vi "CRYUnflatten Calibration 2D.vi"(11 "Flattened Calibration":string) -> (0 "Error?":bool=TRUE, 2 "Calibration Step Out":T1 {"Calibration 2D"."Sens Curve"."Z data" items=["dB", "Lin"]; "Calibration 2D"."Sens Curve"."X data" items=["dB", "Lin"]; "Calibration 2D"."Sens Curve"."Y data" items=["dB", "Lin"]; "Calibration 2D"."Sens Curve"."Z dB ref" format="%.1f"; "Calibration 2D"."Sens Curve"."Z axis" items=["Log", "Lin"]; "Calibration 2D"."Sens Curve"."X dB ref" format="%.1f"; "Calibration 2D"."Sens Curve"."X axis" items=["Log", "Lin"]; "Calibration 2D"."Sens Curve"."Y axis" items=["Log", "Lin"]; "Calibration 2D"."Sens Curve"."Y dB ref" format="%.1f"; "Calibration 2D"."Sens Curve"."Curve"."z" format="%.2f"; "Calibration 2D"."Sens Curve"."Curve"."y" format="%.2f"; "Calibration 2D"."Sens Curve"."Curve"."x" format="%.2f"; "Calibration 2D"."EQ Curve"."Z data" items=["dB", "Lin"]; "Calibration 2D"."EQ Curve"."X data" items=["dB", "Lin"]; "Calibration 2D"."EQ Curve"."Y data" items=["dB", "Lin"]; "Calibration 2D"."EQ Curve"."Z dB ref" format="%.1f"; "Calibration 2D"."EQ Curve"."Z axis" items=["Log", "Lin"]; "Calibration 2D"."EQ Curve"."X dB ref" format="%.1f"; "Calibration 2D"."EQ Curve"."X axis" items=["Log", "Lin"]; "Calibration 2D"."EQ Curve"."Y axis" items=["Log", "Lin"]; "Calibration 2D"."EQ Curve"."Y dB ref" format="%.1f"; "Calibration 2D"."EQ Curve"."Curve"."z" format="%.2f"; "Calibration 2D"."EQ Curve"."Curve"."y" format="%.2f"; "Calibration 2D"."EQ Curve"."Curve"."x" format="%.2f"; "Calibration 2D"."Corr Curve"."Z data" items=["dB", "Lin"]; "Calibration 2D"."Corr Curve"."X data" items=["dB", "Lin"]; "Calibration 2D"."Corr Curve"."Y data" items=["dB", "Lin"]; "Calibration 2D"."Corr Curve"."Z dB ref" format="%.1f"; "Calibration 2D"."Corr Curve"."Z axis" items=["Log", "Lin"]; "Calibration 2D"."Corr Curve"."X dB ref" format="%.1f"; "Calibration 2D"."Corr Curve"."X axis" items=["Log", "Lin"]; "Calibration 2D"."Corr Curve"."Y axis" items=["Log", "Lin"]; "Calibration 2D"."Corr Curve"."Y dB ref" format="%.1f"; "Calibration 2D"."Corr Curve"."Curve"."z" format="%.2f"; "Calibration 2D"."Corr Curve"."Curve"."y" format="%.2f"; "Calibration 2D"."Corr Curve"."Curve"."x" format="%.2f"; "Calibration 2D"."Calibration"."EQ Step size" items=["R10", "R20", "R40", "R80", "User"]; "Calibration 2D"."Calibration"."Corr Step size" items=["R10", "R20", "R40", "R80", "User"]}, 3 "Header info":T5={"Data type"="Data            ", "Version"=1, "Dimensions"=0})   [LabVIEW 2013]
uses:
  Typedef Control/CRYCalibration All Cluster.ctl
  Typedef Control/CRYCalibration 2DCluster.ctl
  Typedef Control/CRYCalibration Cluster.ctl
  Typedef Control/CRYData Cluster.ctl
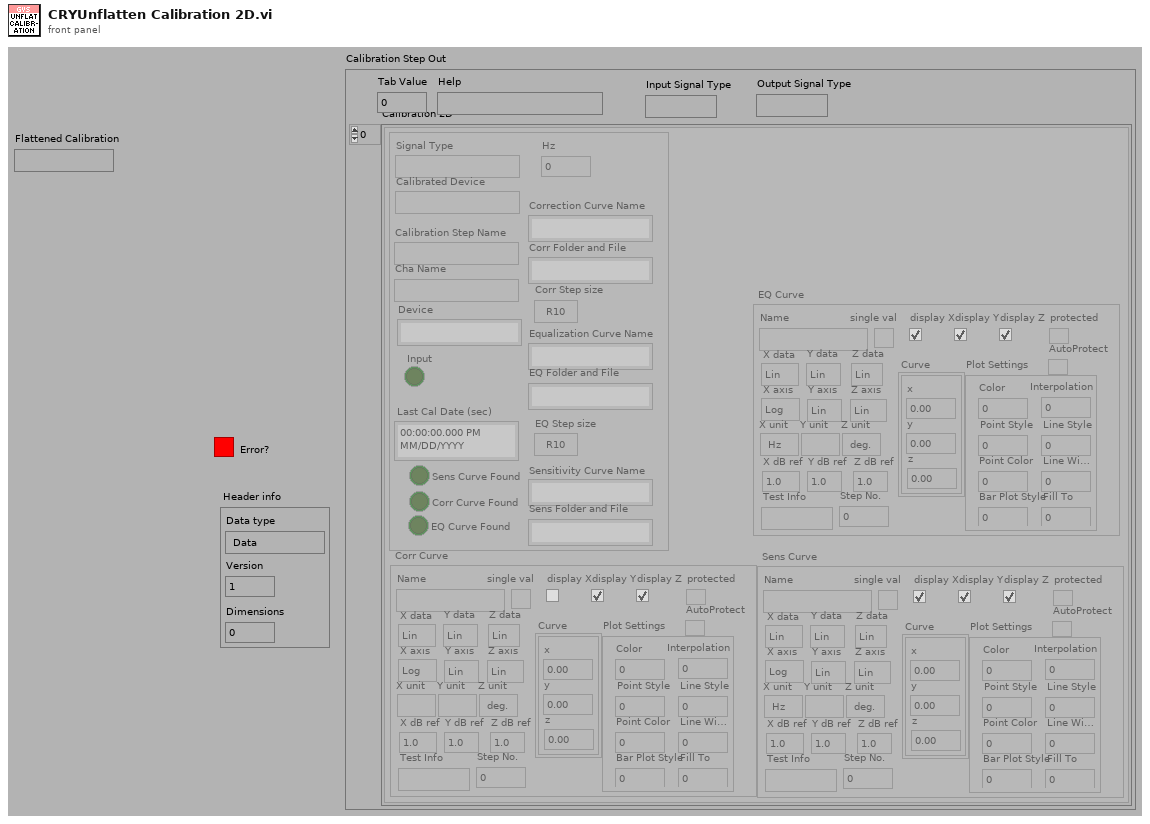
[diagram p1: front panel]
types:
  T1 = typedef "CRYCalibration All Cluster.ctl" = cluster{"Calibration 2D":T2[], "Help":string, "Tab Value":i32, "Input Signal Type":string, "Output Signal Type":string}
  T2 = typedef "CRYCalibration 2DCluster.ctl" = cluster{"Calibration":T3, "Corr Curve":T4, "EQ Curve":T4, "Sens Curve":T4}
  T3 = typedef "CRYCalibration Cluster.ctl" = cluster{"Calibration Step Name":string, "Device":string, "Correction Curve Name":string, "Equalization Curve Name":string, "Sensitivity Curve Name":string, "Corr Folder and File":string, "EQ Folder and File":string, "Sens Folder and File":string, "Corr Step size":u16, "EQ Step size":u16, "Input":bool, "Last Cal Date (sec)":timestamp, "Cha Name":string, "Corr Curve Found":bool, "EQ Curve Found":bool, "Sens Curve Found":bool, "Signal Type":string, "Calibrated Device":string, "Hz":u32}
  T4 = typedef "CRYData Cluster.ctl" = cluster{"Name":string, "Curve":cluster{"x":dbl, "y":dbl, "z":dbl}[], "X data":u16, "Y data":u16, "Z data":u16, "X axis":u16, "Y axis":u16, "Z axis":u16, "X unit":string, "Y unit":string, "Z unit":string, "X dB ref":dbl, "Y dB ref":dbl, "Z dB ref":dbl, "single val":bool, "protected":bool, "display X":bool, "display Y":bool, "display Z":bool, "Test Info":string, "Step No.":i32, "Plot Settings":cluster{"Color":u32, "Interpolation":u8, "Point Style":u8, "Line Style":u8, "Point Color":u32, "Line Width":u8, "Bar Plot Style":u8, "Fill To":i16}, "AutoProtect":bool}
  T5 = cluster{"Data type":string, "Version":u16, "Dimensions":u8}
  T6 = cluster{"Calibration":cluster{"Calibration":cluster{"Calibration Step Name":string, "Last Ch":i32, "Device":string, "Correction Curve Name":string, "Equalization Curve Name":string, "Sensitivity Curve Name":string, "Corr Folder and File":string, "EQ Folder and File":string, "Sens Folder and File":string, "Corr Step size":u16, "EQ Step size":u16, "Input":bool, "Last Cal Date (sec)":timestamp, "Chan Name":string, "Corr Curve Found":bool, "EQ Curve Found":bool, "Sens Curve Found":bool}, "Corr Curve":cluster{"Name":string, "Curve":cluster{"x":dbl, "y":dbl, "z":dbl}[], "X data":u16, "Y data":u16, "Z data":u16, "X axis":u16, "Y axis":u16, "Z axis":u16, "X unit":string, "Y unit":string, "Z unit":string, "X dB ref":dbl, "Y dB ref":dbl, "Z dB ref":dbl, "single val":bool, "protected":bool, "display X":bool, "display Y":bool, "display Z":bool, "Test Info":string, "Step No.":u16, "Plot Settings":cluster{"Color":u32, "Interpolation":u8, "Point Style":u8, "Line Style":u8, "Point Color":u32, "Line Width":u8, "Bar Plot Style":u8, "Fill To":i16}, "AutoProtect":bool}, "EQ Curve":cluster{"Name":string, "Curve":cluster{"x":dbl, "y":dbl, "z":dbl}[], "X data":u16, "Y data":u16, "Z data":u16, "X axis":u16, "Y axis":u16, "Z axis":u16, "X unit":string, "Y unit":string, "Z unit":string, "X dB ref":dbl, "Y dB ref":dbl, "Z dB ref":dbl, "single val":bool, "protected":bool, "display X":bool, "display Y":bool, "display Z":bool, "Test Info":string, "Step No.":u16, "Plot Settings":cluster{"Color":u32, "Interpolation":u8, "Point Style":u8, "Line Style":u8, "Point Color":u32, "Line Width":u8, "Bar Plot Style":u8, "Fill To":i16}, "AutoProtect":bool}, "Sens Curve":cluster{"Name":string, "Curve":cluster{"x":dbl, "y":dbl, "z":dbl}[], "X data":u16, "Y data":u16, "Z data":u16, "X axis":u16, "Y axis":u16, "Z axis":u16, "X unit":string, "Y unit":string, "Z unit":string, "X dB ref":dbl, "Y dB ref":dbl, "Z dB ref":dbl, "single val":bool, "protected":bool, "display X":bool, "display Y":bool, "display Z":bool, "Test Info":string, "Step No.":u16, "Plot Settings":cluster{"Color":u32, "Interpolation":u8, "Point Style":u8, "Line Style":u8, "Point Color":u32, "Line Width":u8, "Bar Plot Style":u8, "Fill To":i16}, "AutoProtect":bool}}[], "Help":string, "Tab Value":i32}
  T7 = cluster{"Calibration 2D":cluster{"Calibration":cluster{"Calibration Step Name":string, "Last Ch":i32, "Device":string, "Correction Curve Name":string, "Equalization Curve Name":string, "Sensitivity Curve Name":string, "Corr Folder and File":string, "EQ Folder and File":string, "Sens Folder and File":string, "Corr Step size":u16, "EQ Step size":u16, "Input":bool, "Last Cal Date (sec)":timestamp, "Cha Name":string, "Corr Curve Found":bool, "EQ Curve Found":bool, "Sens Curve Found":bool}, "Corr Curve":cluster{"Name":string, "Curve":cluster{"x":dbl, "y":dbl, "z":dbl}[], "X data":u16, "Y data":u16, "Z data":u16, "X axis":u16, "Y axis":u16, "Z axis":u16, "X unit":string, "Y unit":string, "Z unit":string, "X dB ref":dbl, "Y dB ref":dbl, "Z dB ref":dbl, "single val":bool, "protected":bool, "display X":bool, "display Y":bool, "display Z":bool, "Test Info":string, "Step No.":i32, "Plot Settings":cluster{"Color":u32, "Interpolation":u8, "Point Style":u8, "Line Style":u8, "Point Color":u32, "Line Width":u8, "Bar Plot Style":u8, "Fill To":i16}, "AutoProtect":bool}, "EQ Curve":cluster{"Name":string, "Curve":cluster{"x":dbl, "y":dbl, "z":dbl}[], "X data":u16, "Y data":u16, "Z data":u16, "X axis":u16, "Y axis":u16, "Z axis":u16, "X unit":string, "Y unit":string, "Z unit":string, "X dB ref":dbl, "Y dB ref":dbl, "Z dB ref":dbl, "single val":bool, "protected":bool, "display X":bool, "display Y":bool, "display Z":bool, "Test Info":string, "Step No.":i32, "Plot Settings":cluster{"Color":u32, "Interpolation":u8, "Point Style":u8, "Line Style":u8, "Point Color":u32, "Line Width":u8, "Bar Plot Style":u8, "Fill To":i16}, "AutoProtect":bool}, "Sens Curve":cluster{"Name":string, "Curve":cluster{"x":dbl, "y":dbl, "z":dbl}[], "X data":u16, "Y data":u16, "Z data":u16, "X axis":u16, "Y axis":u16, "Z axis":u16, "X unit":string, "Y unit":string, "Z unit":string, "X dB ref":dbl, "Y dB ref":dbl, "Z dB ref":dbl, "single val":bool, "protected":bool, "display X":bool, "display Y":bool, "display Z":bool, "Test Info":string, "Step No.":i32, "Plot Settings":cluster{"Color":u32, "Interpolation":u8, "Point Style":u8, "Line Style":u8, "Point Color":u32, "Line Width":u8, "Bar Plot Style":u8, "Fill To":i16}, "AutoProtect":bool}}[], "Help":string, "Tab Value":i32}
  T8 = cluster{"unsigned byte array[0]":u8, "unsigned byte array[1]":u8, "unsigned byte array[2]":u8}
  T9 = cluster{"Calibration":cluster{"Calibration Step Name":string, "Last Ch":i32, "Device":string, "Correction Curve Name":string, "Equalization Curve Name":string, "Sensitivity Curve Name":string, "Corr Folder and File":string, "EQ Folder and File":string, "Sens Folder and File":string, "Corr Step size":u16, "EQ Step size":u16, "Input":bool, "Last Cal Date (sec)":timestamp, "Chan Name":string, "Corr Curve Found":bool, "EQ Curve Found":bool, "Sens Curve Found":bool}, "Corr Curve":cluster{"Name":string, "Curve":cluster{"x":dbl, "y":dbl, "z":dbl}[], "X data":u16, "Y data":u16, "Z data":u16, "X axis":u16, "Y axis":u16, "Z axis":u16, "X unit":string, "Y unit":string, "Z unit":string, "X dB ref":dbl, "Y dB ref":dbl, "Z dB ref":dbl, "single val":bool, "protected":bool, "display X":bool, "display Y":bool, "display Z":bool, "Test Info":string, "Step No.":u16, "Plot Settings":cluster{"Color":u32, "Interpolation":u8, "Point Style":u8, "Line Style":u8, "Point Color":u32, "Line Width":u8, "Bar Plot Style":u8, "Fill To":i16}, "AutoProtect":bool}, "EQ Curve":cluster{"Name":string, "Curve":cluster{"x":dbl, "y":dbl, "z":dbl}[], "X data":u16, "Y data":u16, "Z data":u16, "X axis":u16, "Y axis":u16, "Z axis":u16, "X unit":string, "Y unit":string, "Z unit":string, "X dB ref":dbl, "Y dB ref":dbl, "Z dB ref":dbl, "single val":bool, "protected":bool, "display X":bool, "display Y":bool, "display Z":bool, "Test Info":string, "Step No.":u16, "Plot Settings":cluster{"Color":u32, "Interpolation":u8, "Point Style":u8, "Line Style":u8, "Point Color":u32, "Line Width":u8, "Bar Plot Style":u8, "Fill To":i16}, "AutoProtect":bool}, "Sens Curve":cluster{"Name":string, "Curve":cluster{"x":dbl, "y":dbl, "z":dbl}[], "X data":u16, "Y data":u16, "Z data":u16, "X axis":u16, "Y axis":u16, "Z axis":u16, "X unit":string, "Y unit":string, "Z unit":string, "X dB ref":dbl, "Y dB ref":dbl, "Z dB ref":dbl, "single val":bool, "protected":bool, "display X":bool, "display Y":bool, "display Z":bool, "Test Info":string, "Step No.":u16, "Plot Settings":cluster{"Color":u32, "Interpolation":u8, "Point Style":u8, "Line Style":u8, "Point Color":u32, "Line Width":u8, "Bar Plot Style":u8, "Fill To":i16}, "AutoProtect":bool}}[]
  T10 = cluster{"Calibration Step Name":string, "Last Ch":i32, "Device":string, "Correction Curve Name":string, "Equalization Curve Name":string, "Sensitivity Curve Name":string, "Corr Folder and File":string, "EQ Folder and File":string, "Sens Folder and File":string, "Corr Step size":u16, "EQ Step size":u16, "Input":bool, "Last Cal Date (sec)":timestamp, "Chan Name":string, "Corr Curve Found":bool, "EQ Curve Found":bool, "Sens Curve Found":bool}
  T11 = cluster{"Name":string, "Curve":cluster{"x":dbl, "y":dbl, "z":dbl}[], "X data":u16, "Y data":u16, "Z data":u16, "X axis":u16, "Y axis":u16, "Z axis":u16, "X unit":string, "Y unit":string, "Z unit":string, "X dB ref":dbl, "Y dB ref":dbl, "Z dB ref":dbl, "single val":bool, "protected":bool, "display X":bool, "display Y":bool, "display Z":bool, "Test Info":string, "Step No.":u16, "Plot Settings":cluster{"Color":u32, "Interpolation":u8, "Point Style":u8, "Line Style":u8, "Point Color":u32, "Line Width":u8, "Bar Plot Style":u8, "Fill To":i16}, "AutoProtect":bool}
  T12 = cluster{"Calibration":cluster{"Calibration Step Name":string, "Last Ch":i32, "Device":string, "Correction Curve Name":string, "Equalization Curve Name":string, "Sensitivity Curve Name":string, "Corr Folder and File":string, "EQ Folder and File":string, "Sens Folder and File":string, "Corr Step size":u16, "EQ Step size":u16, "Input":bool, "Last Cal Date (sec)":timestamp, "Cha Name":string, "Corr Curve Found":bool, "EQ Curve Found":bool, "Sens Curve Found":bool}, "Corr Curve":cluster{"Name":string, "Curve":cluster{"x":dbl, "y":dbl, "z":dbl}[], "X data":u16, "Y data":u16, "Z data":u16, "X axis":u16, "Y axis":u16, "Z axis":u16, "X unit":string, "Y unit":string, "Z unit":string, "X dB ref":dbl, "Y dB ref":dbl, "Z dB ref":dbl, "single val":bool, "protected":bool, "display X":bool, "display Y":bool, "display Z":bool, "Test Info":string, "Step No.":i32, "Plot Settings":cluster{"Color":u32, "Interpolation":u8, "Point Style":u8, "Line Style":u8, "Point Color":u32, "Line Width":u8, "Bar Plot Style":u8, "Fill To":i16}, "AutoProtect":bool}, "EQ Curve":cluster{"Name":string, "Curve":cluster{"x":dbl, "y":dbl, "z":dbl}[], "X data":u16, "Y data":u16, "Z data":u16, "X axis":u16, "Y axis":u16, "Z axis":u16, "X unit":string, "Y unit":string, "Z unit":string, "X dB ref":dbl, "Y dB ref":dbl, "Z dB ref":dbl, "single val":bool, "protected":bool, "display X":bool, "display Y":bool, "display Z":bool, "Test Info":string, "Step No.":i32, "Plot Settings":cluster{"Color":u32, "Interpolation":u8, "Point Style":u8, "Line Style":u8, "Point Color":u32, "Line Width":u8, "Bar Plot Style":u8, "Fill To":i16}, "AutoProtect":bool}, "Sens Curve":cluster{"Name":string, "Curve":cluster{"x":dbl, "y":dbl, "z":dbl}[], "X data":u16, "Y data":u16, "Z data":u16, "X axis":u16, "Y axis":u16, "Z axis":u16, "X unit":string, "Y unit":string, "Z unit":string, "X dB ref":dbl, "Y dB ref":dbl, "Z dB ref":dbl, "single val":bool, "protected":bool, "display X":bool, "display Y":bool, "display Z":bool, "Test Info":string, "Step No.":i32, "Plot Settings":cluster{"Color":u32, "Interpolation":u8, "Point Style":u8, "Line Style":u8, "Point Color":u32, "Line Width":u8, "Bar Plot Style":u8, "Fill To":i16}, "AutoProtect":bool}}[]
  T13 = cluster{"Calibration Step Name":string, "Last Ch":i32, "Device":string, "Correction Curve Name":string, "Equalization Curve Name":string, "Sensitivity Curve Name":string, "Corr Folder and File":string, "EQ Folder and File":string, "Sens Folder and File":string, "Corr Step size":u16, "EQ Step size":u16, "Input":bool, "Last Cal Date (sec)":timestamp, "Cha Name":string, "Corr Curve Found":bool, "EQ Curve Found":bool, "Sens Curve Found":bool}
  T14 = cluster{"Name":string, "Curve":cluster{"x":dbl, "y":dbl, "z":dbl}[], "X data":u16, "Y data":u16, "Z data":u16, "X axis":u16, "Y axis":u16, "Z axis":u16, "X unit":string, "Y unit":string, "Z unit":string, "X dB ref":dbl, "Y dB ref":dbl, "Z dB ref":dbl, "single val":bool, "protected":bool, "display X":bool, "display Y":bool, "display Z":bool, "Test Info":string, "Step No.":i32, "Plot Settings":cluster{"Color":u32, "Interpolation":u8, "Point Style":u8, "Line Style":u8, "Point Color":u32, "Line Width":u8, "Bar Plot Style":u8, "Fill To":i16}, "AutoProtect":bool}
  T15 = cluster{"substring":string, u16, "unsigned byte array[2]":u8}
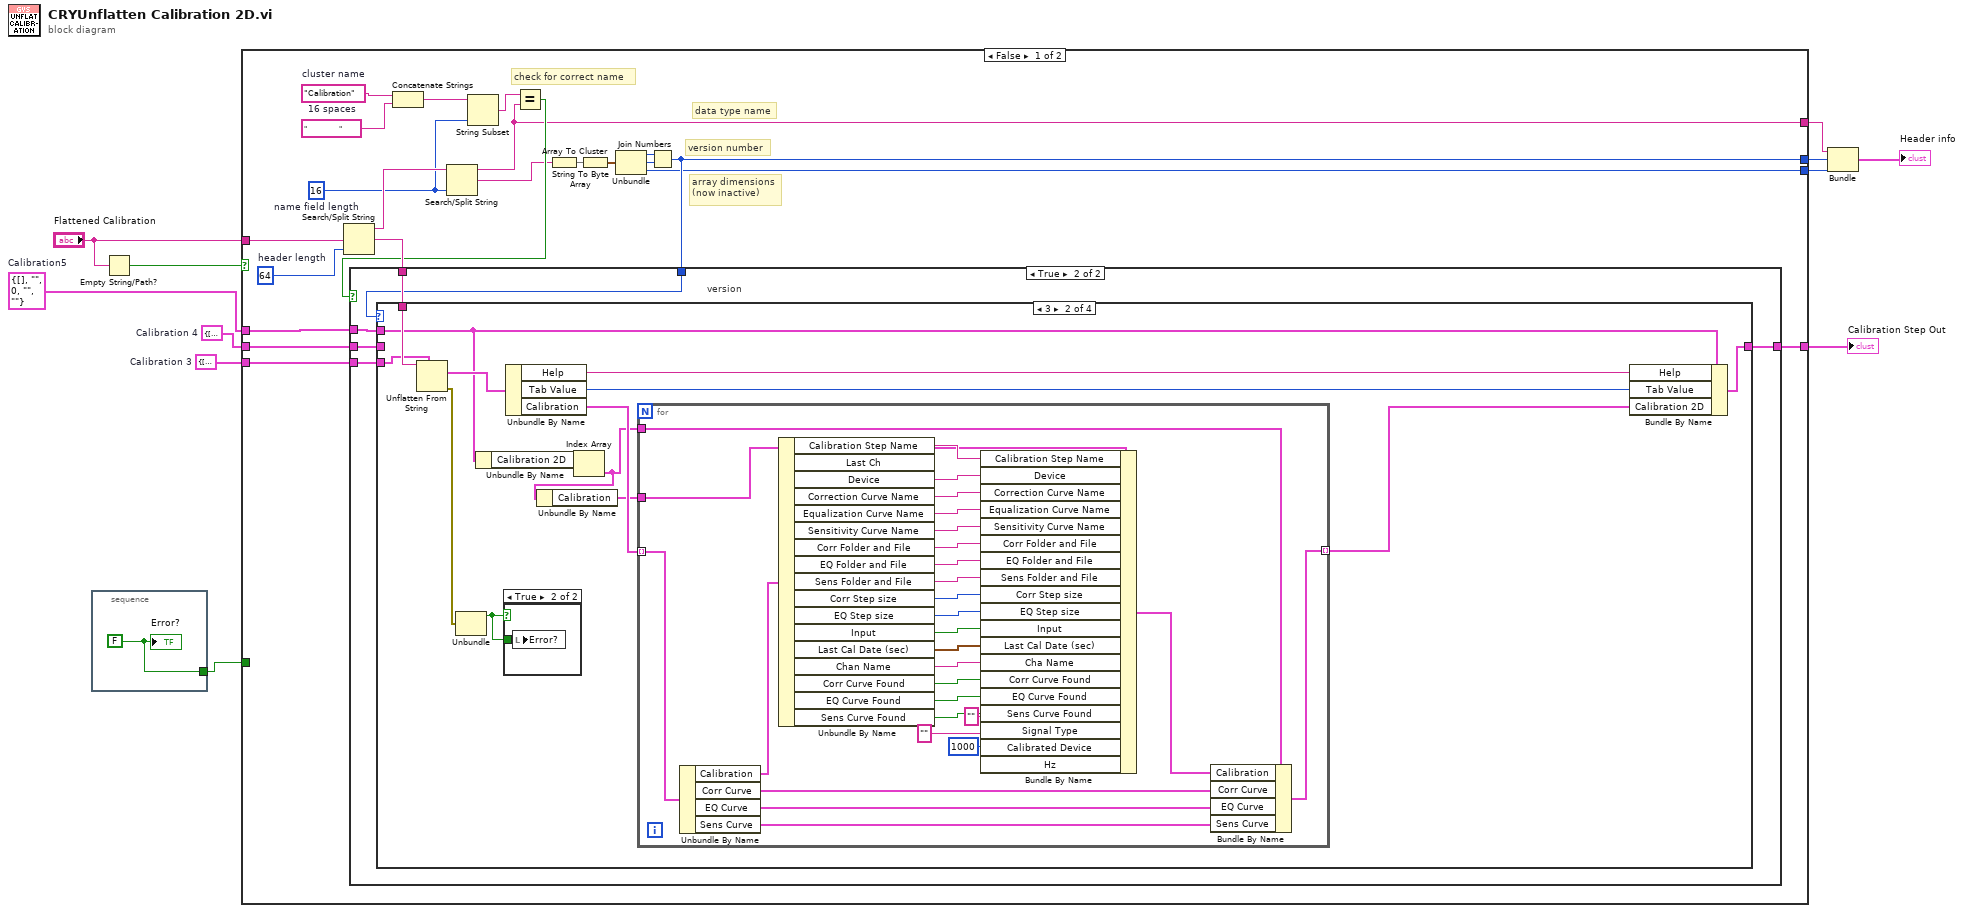
[diagram p0: block diagram]
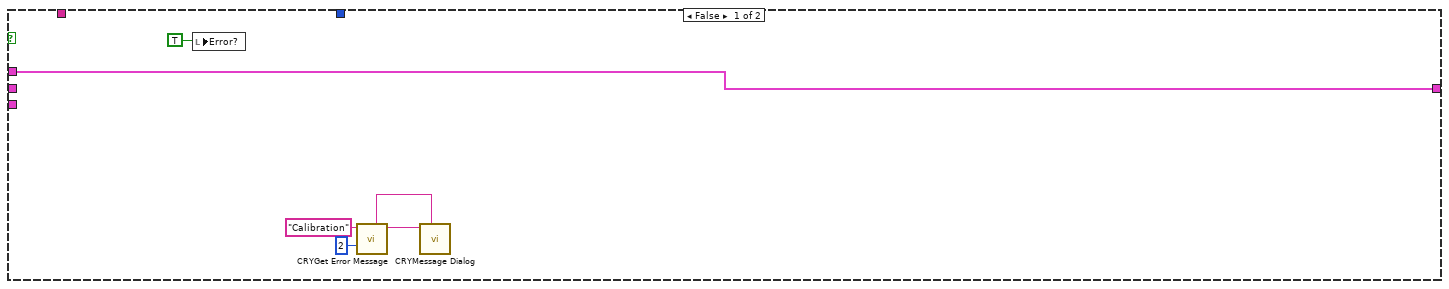
[diagram p2: hidden frame]
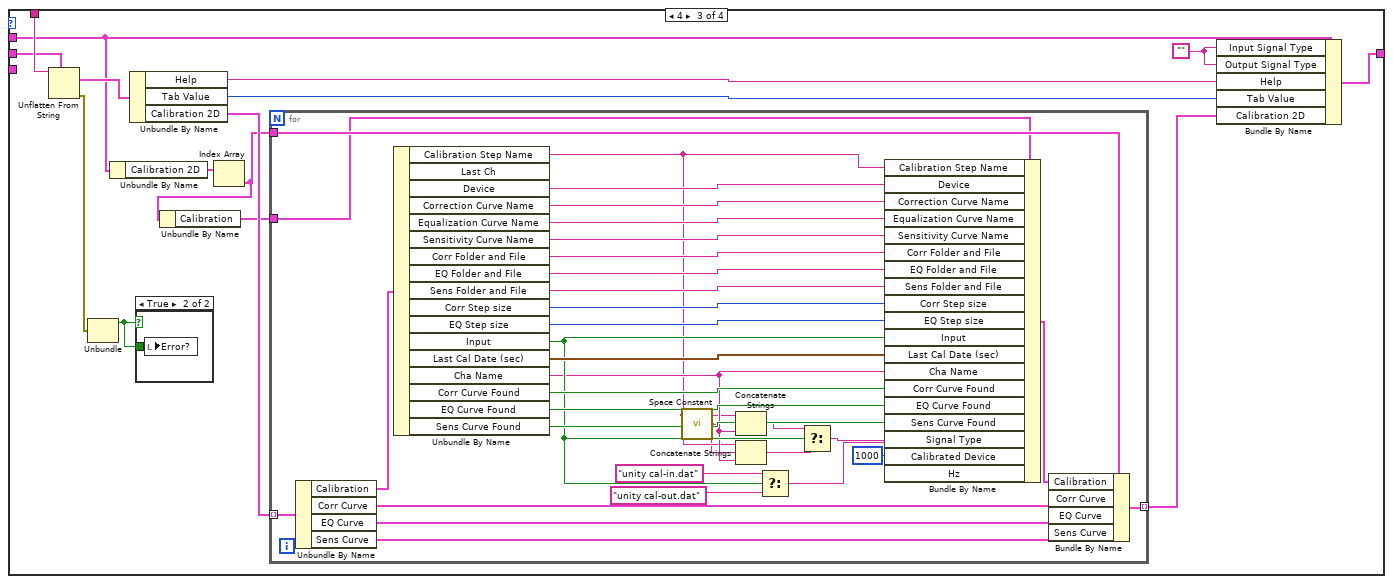
[diagram p5: hidden frame]
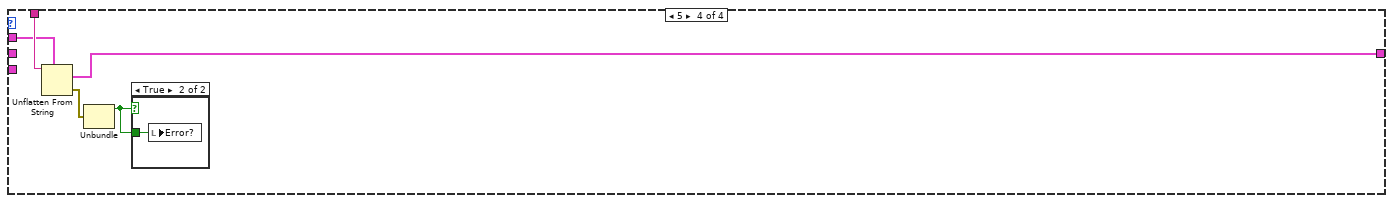
[diagram p7: hidden frame]
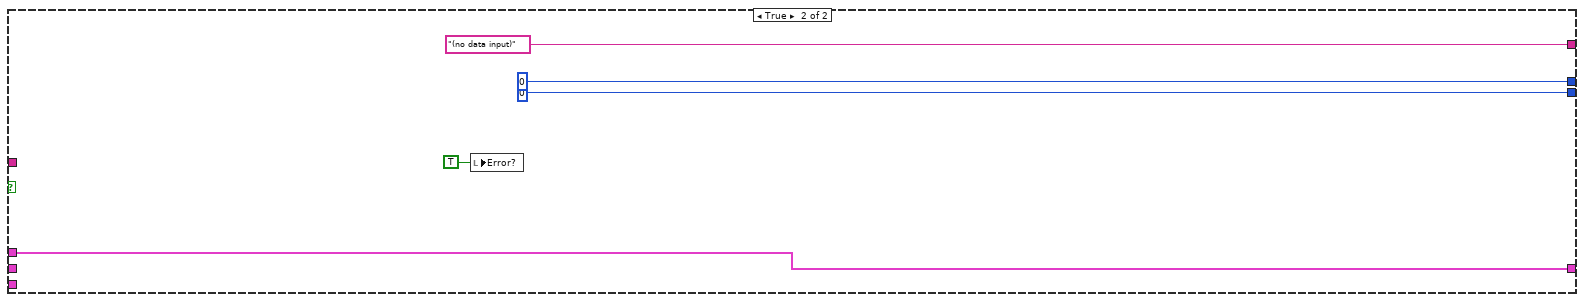
[diagram p9: hidden frame]
diagram:
  w2 = T1 {"Calibration 2D"=[], "Help"="", "Tab Value"=0, "Input Signal Type"="", "Output Signal Type"=""}  # Calibration5
  w3 = T6 {"Calibration"=[], "Help"="", "Tab Value"=0}  # Calibration 3
  w1 = T7 {"Calibration 2D"=[], "Help"="", "Tab Value"=0}  # Calibration 4
  n1 = stacked-sequence {
    tunnel: [w12] -> w5
    frame #0 {
      w12 = FALSE
      "Error?" <- w12
    }
  }
  n2 = Empty String/Path?(string/path="Flattened Calibration") -> (empty?=w10:bool)
  n3 = case shown="False" w10 {
    tunnel: "Flattened Calibration" -> [w34 _]
    tunnel: [w26 u16 0] -> w8
    tunnel: [w19 u8 0] -> w9
    tunnel: [w20 "(no data input)" ("substring")] -> w7
    tunnel: w5 -> [_ _]
    tunnel: [w18 w146] -> w4
    tunnel: w2 -> [w17 w146]
    tunnel: w3 -> [w14 _]
    tunnel: w1 -> [w13 _]
    frame False {
      w15 = 64  # header length
      w24 = "                "  # 16 spaces
      w16 = "Calibration"  # cluster name
      w22 = 16  # name field length
      # "check for correct name"
      # "array dimensions\n(now inactive)"
      # "version number"
      # "data type name"
      n4 = Search/Split String(string=w34, offset (0)=w15) -> (substring before match=w28:string, match + rest of string=w29:string)  [unwired: 2 out]
      n5 = Concatenate Strings(w16, w24) -> (w23:string)
      n6 = Search/Split String(string=w28, offset (0)=w22) -> (substring before match=w20:string, match + rest of string=w25:string)  [unwired: 2 out]
      n7 = String Subset(string=w23, length (rest)=w22) -> (substring=w21:string)  [unwired: 1 out]
      n8 = Equal?(x=w21, y=w20) -> (x = y?=w27:bool)
      n9 = String To Byte Array(string=w25) -> (unsigned byte array=w33:u8[])
      n10 = Array To Cluster(array=w33) -> (cluster=w32:T8)
      n11 = Unbundle(w32) -> ("unsigned byte array[0]"=w31:u8, "unsigned byte array[1]"=w30:u8, "unsigned byte array[2]"=w19:u8)
      n12 = Join Numbers(hi=w31, lo=w30) -> ((hi.lo)=w26:u16)
      n13 = case shown="True" w27 {
        tunnel: w29 -> [_ w46]
        tunnel: w26 -> [_ w45]
        tunnel: [w39 w44] -> w18
        tunnel: w17 -> [w39 w43]
        tunnel: w14 -> [_ w42]
        tunnel: w13 -> [_ w41]
        frame False {
          n14 = local write "Error?"(TRUE) -> ()
          n15 = call "CRYGet Error Message.vi"("Error No"=2, "Kind"="Calibration") -> ("Message"=w36:string, "Window Title"=w35:string)  [unwired: 4 in, 4 out]
          n16 = call "CRYMessage Dialog.vi"("Window Title"=w35, "Message Content"=w36) -> ()  [unwired: 8 in, 2 out]
        }
        frame True {
          n17 = case "version" shown="3" w45 {
            tunnel: w46 -> [_ w59 w103 w144]
            tunnel: [w47 w58 w102 w140] -> w44
            tunnel: w43 -> [w47 w52 w97 w141]
            tunnel: w42 -> [_ w57 _ _]
            tunnel: w41 -> [_ _ w94 _]
            frame 0, Default {
            }
            frame 3 {
              n18 = Unflatten From String(type=w57, binary string=w59) -> (value=w56:T6, error out=w60:errorcluster)  [unwired: 1 in, 3 out]
              n19 = Unbundle(w60) -> ("status"=w61:bool)  [unwired: 2 out]
              n20 = Unbundle By Name(w52) -> ("Calibration 2D"=w50:T2[])
              n21 = case shown="True" w61 {
                tunnel: w61 -> [_ w90]
                frame False {
                }
                frame True {
                  n22 = local write "Error?"(w90) -> ()
                }
              }
              n23 = Unbundle By Name(w56) -> ("Help"=w55:string, "Tab Value"=w54:i32, "Calibration"=w53:T9)
              n24 = Index Array(array=w50) -> (element=w49:T2)  [unwired: 1 in]
              n25 = Unbundle By Name(w49) -> ("Calibration"=w48:T3)
              n26 = for {
                tunnel: w53 -> [w89] mode=indexing
                tunnel: w49 -> [w81]
                tunnel: [w85] -> w51 mode=indexing
                tunnel: w48 -> [w62]
                n27 = Unbundle By Name(w89) -> ("Calibration"=w82:T10, "Corr Curve"=w88:T11, "EQ Curve"=w87:T11, "Sens Curve"=w86:T11)
                n28 = Unbundle By Name(w82) -> ("Calibration Step Name"=w79:string, "Device"=w77:string, "Correction Curve Name"=w76:string, "Equalization Curve Name"=w75:string, "Sensitivity Curve Name"=w74:string, "Corr Folder and File"=w73:string, "EQ Folder and File"=w72:string, "Sens Folder and File"=w71:string, "Corr Step size"=w70:u16, "EQ Step size"=w69:u16, "Input"=w68:bool, "Last Cal Date (sec)"=w67:timestamp, "Chan Name"=w66:string, "Corr Curve Found"=w65:bool, "EQ Curve Found"=w64:bool, "Sens Curve Found"=w80:bool)  [unwired: 1 out]
                n29 = Bundle By Name(cluster=w62, "Calibration Step Name"=w79, "Device"=w77, "Correction Curve Name"=w76, "Equalization Curve Name"=w75, "Sensitivity Curve Name"=w74, "Corr Folder and File"=w73, "EQ Folder and File"=w72, "Sens Folder and File"=w71, "Corr Step size"=w70, "EQ Step size"=w69, "Input"=w68, "Last Cal Date (sec)"=w67, "Cha Name"=w66, "Corr Curve Found"=w65, "EQ Curve Found"=w64, "Sens Curve Found"=w80, "Signal Type"="", "Calibrated Device"="", "Hz"=u32 1000) -> (w78:T3)
                n30 = Bundle By Name(cluster=w81, "Calibration"=w78, "Corr Curve"=w88, "EQ Curve"=w87, "Sens Curve"=w86) -> (w85:T2)
              }
              n31 = Bundle By Name(cluster=w52, "Help"=w55, "Tab Value"=w54, "Calibration 2D"=w51) -> (w58:T1)
            }
            frame 4 {
              w91 = "" ("Input Signal Type")
              n32 = Unflatten From String(type=w94, binary string=w103) -> (value=w101:T7, error out=w104:errorcluster)  [unwired: 1 in, 3 out]
              n33 = Unbundle(w104) -> ("status"=w105:bool)  [unwired: 2 out]
              n34 = Unbundle By Name(w97) -> ("Calibration 2D"=w95:T2[])
              n35 = Unbundle By Name(w101) -> ("Help"=w100:string, "Tab Value"=w99:i32, "Calibration 2D"=w98:T12)
              n36 = case shown="True" w105 {
                tunnel: w105 -> [_ w139]
                frame False {
                }
                frame True {
                  n37 = local write "Error?"(w139) -> ()
                }
              }
              n38 = Index Array(array=w95) -> (element=w93:T2)  [unwired: 1 in]
              n39 = Unbundle By Name(w93) -> ("Calibration"=w92:T3)
              n40 = for {
                tunnel: w98 -> [w138] mode=indexing
                tunnel: w93 -> [w131]
                tunnel: [w134] -> w96 mode=indexing
                tunnel: w92 -> [w116]
                n41 = Unbundle By Name(w138) -> ("Calibration"=w133:T13, "Corr Curve"=w137:T14, "EQ Curve"=w136:T14, "Sens Curve"=w135:T14)
                n42 = Unbundle By Name(w133) -> ("Calibration Step Name"=w107:string, "Device"=w130:string, "Correction Curve Name"=w129:string, "Equalization Curve Name"=w128:string, "Sensitivity Curve Name"=w127:string, "Corr Folder and File"=w126:string, "EQ Folder and File"=w125:string, "Sens Folder and File"=w124:string, "Corr Step size"=w123:u16, "EQ Step size"=w122:u16, "Input"=w114:bool, "Last Cal Date (sec)"=w121:timestamp, "Cha Name"=w108:string, "Corr Curve Found"=w120:bool, "EQ Curve Found"=w119:bool, "Sens Curve Found"=w118:bool)  [unwired: 1 out]
                n43 = call <vilib>:"Space Constant.vi"() -> ("String"=w106:string)
                n44 = Concatenate Strings(w107, w106, w108) -> (w109:string)
                n45 = Concatenate Strings(w107, w106, w108) -> (w110:string)
                n46 = Select(t="unity cal-in.dat" ("Calibrated Device"), s=w114, f="unity cal-out.dat" ("Calibrated Device")) -> (s? t:f=w111:string)
                n47 = Select(t=w109, s=w114, f=w110) -> (s? t:f=w115:string)
                n48 = Bundle By Name(cluster=w116, "Calibration Step Name"=w107, "Device"=w130, "Correction Curve Name"=w129, "Equalization Curve Name"=w128, "Sensitivity Curve Name"=w127, "Corr Folder and File"=w126, "EQ Folder and File"=w125, "Sens Folder and File"=w124, "Corr Step size"=w123, "EQ Step size"=w122, "Input"=w114, "Last Cal Date (sec)"=w121, "Cha Name"=w108, "Corr Curve Found"=w120, "EQ Curve Found"=w119, "Sens Curve Found"=w118, "Signal Type"=w115, "Calibrated Device"=w111, "Hz"=u32 1000) -> (w132:T3)
                n49 = Bundle By Name(cluster=w131, "Calibration"=w132, "Corr Curve"=w137, "EQ Curve"=w136, "Sens Curve"=w135) -> (w134:T2)
              }
              n50 = Bundle By Name(cluster=w97, "Input Signal Type"=w91, "Output Signal Type"=w91, "Help"=w100, "Tab Value"=w99, "Calibration 2D"=w96) -> (w102:T1)
            }
            frame 5 {
              n51 = Unflatten From String(type=w141, binary string=w144) -> (value=w140:T1, error out=w142:errorcluster)  [unwired: 1 in, 3 out]
              n52 = Unbundle(w142) -> ("status"=w143:bool)  [unwired: 2 out]
              n53 = case shown="True" w143 {
                tunnel: w143 -> [_ w145]
                frame False {
                }
                frame True {
                  n54 = local write "Error?"(w145) -> ()
                }
              }
            }
          }
        }
      }
    }
    frame True {
      n55 = local write "Error?"(TRUE ("Error?")) -> ()
    }
  }
  "Calibration Step Out" <- w4
  n56 = Bundle("substring"=w7, w8, "unsigned byte array[2]"=w9) -> (→"Header info":T15)  [unwired: 1 out]
